vi "Initialize MM Network.vi"(7 "Net Adress":string, 8 "error in (no error)":errorcluster, 11 "Sensor Engine Datas in":T1[](array[typedef]) {"MM Frames"."payload" format="%x"; "MM Frames"."timestamp" format="%<%.7X\n%x>T"; "MM Frames"."type" items=["FlexRay Data"=32, "FlexRay Null"=33, "FlexRay Symbol"=34, "Log Trigger"=225, "Start Trigger"=226]; "MM Frames"."cycle count" max=63 step=1}) -> (0 "error out":errorcluster, 3 "Sensor Engine Datas out":T1[](array[typedef]) {"MM Frames"."payload" format="%x"; "MM Frames"."timestamp" format="%<%.7X\n%x>T"; "MM Frames"."type" items=["FlexRay Data"=32, "FlexRay Null"=33, "FlexRay Symbol"=34, "Log Trigger"=225, "Start Trigger"=226]; "MM Frames"."cycle count" max=63 step=1})   [LabVIEW 2018, in "MM.lvlib"]
uses:
  MM.lvlib
  Sensor Engine Data.ctl
  Shared/Protocol.ctl
  Shared/Sensor Name.ctl
  <vilib>/xnet/xnet.llb/XNET Frame FlexRay.ctl
  <vilib>/xnet/xnet.llb/XNET Frame Type FlexRay.ctl
  Engine/Vires VTD Engine.lvlib
  Shared/Vires VTD Shared.lvlib
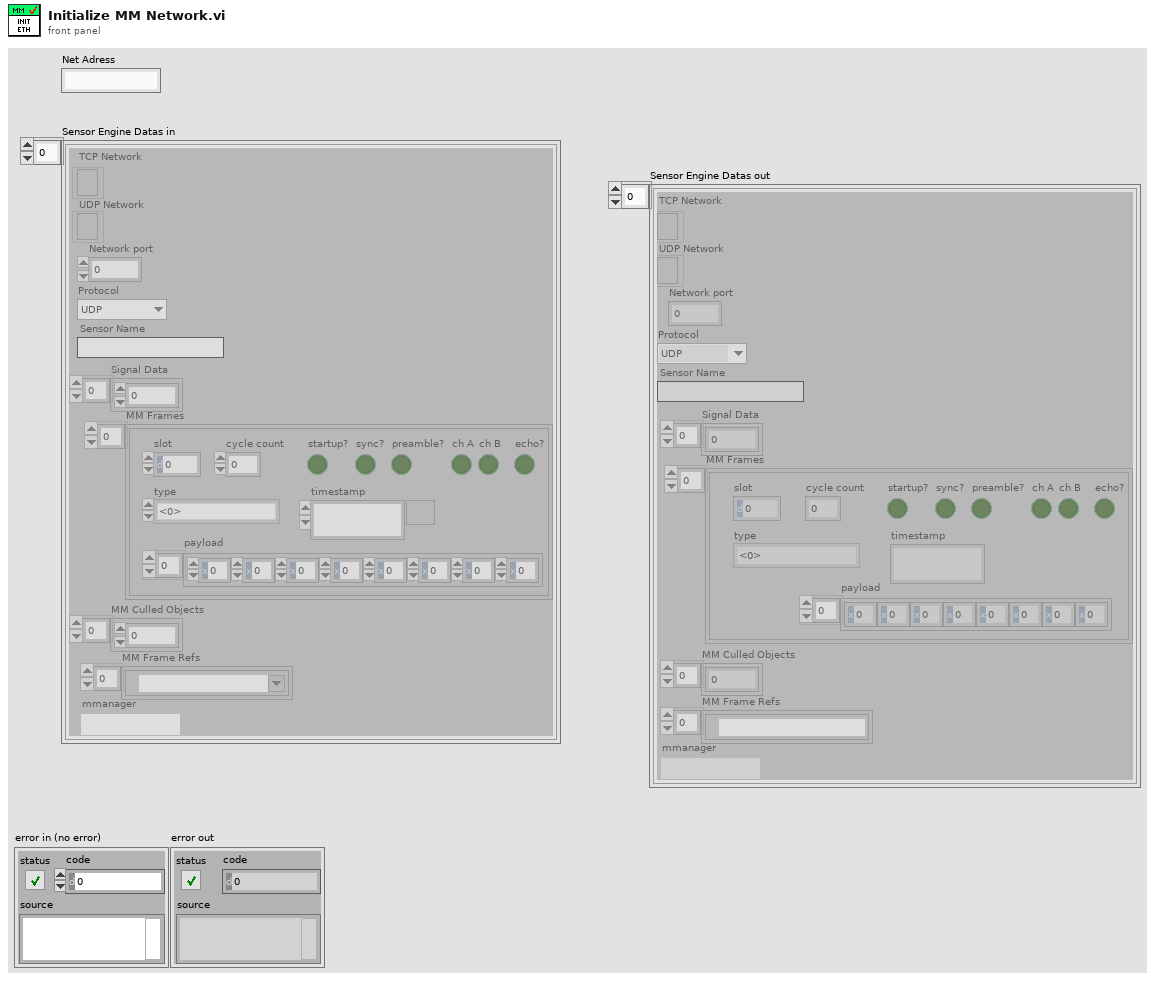
[diagram p1: front panel]
types:
  T1 = typedef "MM.lvlib/Sensor Engine Data.ctl" = cluster{"TCP Network":refnum<k5>, "UDP Network":refnum<k16>, "Network port":i32, "Protocol":T2, "Sensor Name":T3, "Signal Data":dbl[], "MM Frames":T4[], "MM Culled Objects":i32[], "MM Frame Refs":refnum<k21>[], "mmanager":path}
  T2 = typedef "Vires VTD Shared.lvlib/Protocol.ctl" = enum16{"UDP", "TCP"}
  T3 = typedef "Vires VTD Shared.lvlib/Sensor Name.ctl" = string
  T4 = typedef "XNET Frame FlexRay.ctl" = cluster{"timestamp":timestamp, "payload":u8[], "slot":u16, "type":T5, "cycle count":u8, "startup?":bool, "sync?":bool, "preamble?":bool, "ch A":bool, "ch B":bool, "echo?":bool}
  T5 = typedef "XNET Frame Type FlexRay.ctl" = u8
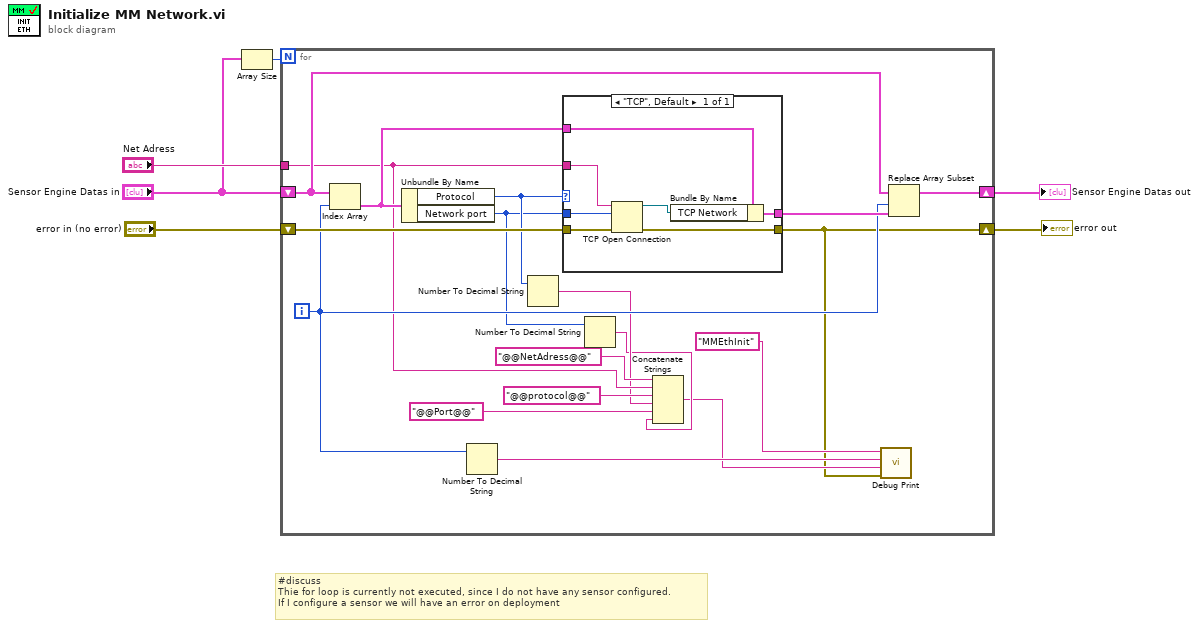
[diagram p0: block diagram]
diagram:
  # "#discuss\nThie for loop is currently not executed, since I do not have any sensor configured.\nIf I configure a sensor we will have an error on deployment"
  n1 = Array Size(array="Sensor Engine Datas in") -> (size(s)=w2:i32)
  n2 = for {
    N: w2 -> [_]
    tunnel: "Net Adress" -> [w13]
    shift-right: [w7] -> w4
    shift-left: "error in (no error)" -> [w24]
    shift-right: [w22] -> w3
    shift-left: "Sensor Engine Datas in" -> [w23]
    i -> [w18]
    n3 = Index Array(array=w23, index=w18) -> (element=w21:T1)
    n4 = Unbundle By Name(w21) -> ("Protocol"=w15:T2, "Network port"=w10:i32)
    n5 = Number To Decimal String(number=w18) -> (decimal integer string=w17:string)  [unwired: 1 in]
    n6 = Number To Decimal String(number=w15) -> (decimal integer string=w12:string)  [unwired: 1 in]
    n7 = case shown="\"TCP\", Default" w15 {
      tunnel: w13 -> [w31]
      tunnel: w10 -> [w30]
      tunnel: w24 -> [w29]
      tunnel: [w28] -> w7
      tunnel: w21 -> [w26]
      tunnel: [w25] -> w20
      frame "TCP", Default {
        n8 = TCP Open Connection(address=w31, remote port or service name=w30, error in (no error)=w29) -> (connection ID=w27:refnum<k5>, error out=w28:errorcluster)  [unwired: 2 in]
        n9 = Bundle By Name(cluster=w26, "TCP Network"=w27) -> (w25:T1)
      }
    }
    n10 = Number To Decimal String(number=w10) -> (decimal integer string=w9:string)  [unwired: 1 in]
    n11 = Concatenate Strings("@@NetAdress@@" ("string"), w13, "@@protocol@@" ("string"), w12, "@@Port@@" ("string"), w9) -> (w8:string)
    n12 = call "Debug Print.vi"("error out"=w7, "comment"=w8, "Index"=w17, "Module"="MMEthInit") -> ()  [unwired: 8 in]
    n13 = Replace Array Subset(array=w23, new element=w20, index=w18) -> (w22:T1[])
  }
  "error out" <- w4
  "Sensor Engine Datas out" <- w3
